vi "Put Object from file (Multipart).vi"(4 "Region":T1, 6 "Chunk size (kB)":i32=5120 min=5120, 7 "Request Parameters":T3={"Content Type"="binary/octet-stream", "ACL"=enum."private", "Storage Class"=enum."STANDARD", "User Metadata"=[]}, 8 "error in (no error)":errorcluster, 9 "Bucket":string, 10 "Object Path":string, 11 "Local file path":path) -> (0 "error out":errorcluster, 2 "Version ID":string, 3 "CompleteMultipartUploadResult":T2)   [LabVIEW 2015, in "LV Interface for Amazon S3.lvlib"]
doc: "This operation <B>uploads an object from a file</B> to a bucket <B>in multiple parts</B>. You can <B>set Chunk size (kB) to limit memory usage</B> of the operation."
uses:
  LV Interface for Amazon S3.lvlib
  Typedefs/AMZ_S3_API_POST Multipart Object Request Parameters.ctl
  Typedefs/AMZ_S3_ACL.ctl
  Typedefs/AMZ_S3_Storage Class.ctl
  Typedefs/AMZ_S3_Object Metadata.ctl
  Typedefs/AMZ_S3_API_CompleteMultipartUploadResult.ctl
  Typedefs/AMZ_S3_LocationConstraint.ctl
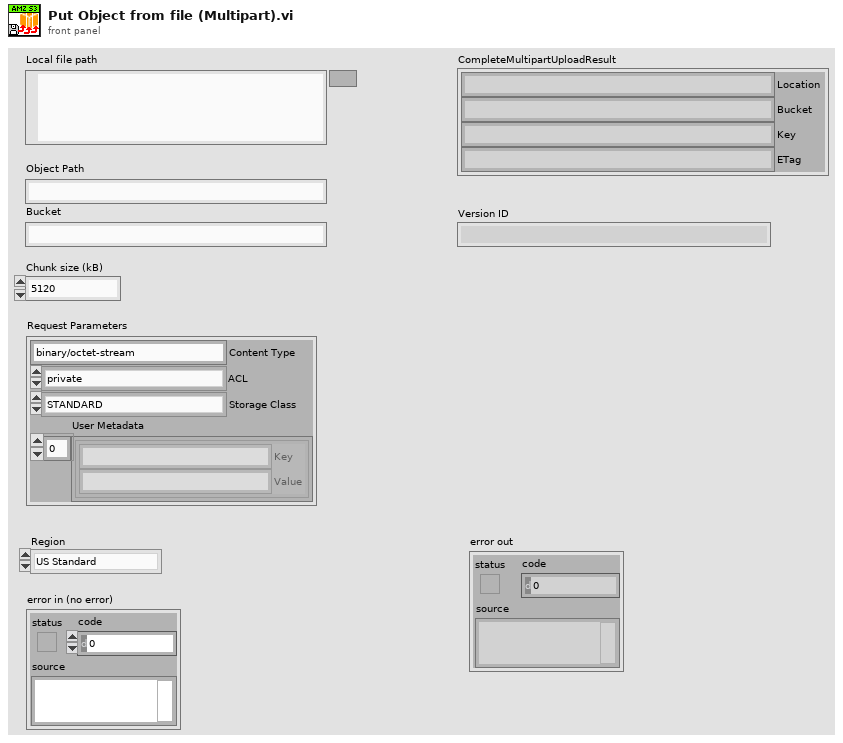
[diagram p1: front panel]
types:
  T1 = typedef "LV Interface for Amazon S3.lvlib/AMZ_S3_LocationConstraint.ctl" = enum16{"US Standard", "us-east-2", "us-west-1", "us-west-2", "ap-northeast-1", "ap-northeast-2", "ap-southeast-1", "ap-southeast-2", "ca-central-1", "eu-central-1", "eu-west-1", "eu-west-2", "sa-east-1"}
  T2 = typedef "LV Interface for Amazon S3.lvlib/AMZ_S3_API_CompleteMultipartUploadResult.ctl" = cluster{"Location":string, "Bucket":string, "Key":string, "ETag":string}
  T3 = typedef "LV Interface for Amazon S3.lvlib/AMZ_S3_API_POST Multipart Object Request Parameters.ctl" = cluster{"Content Type":string, "ACL":T4, "Storage Class":T5, "User Metadata":T6[]}
  T4 = typedef "LV Interface for Amazon S3.lvlib/AMZ_S3_ACL.ctl" = enum16{"private", "public-read", "public-read-write", "aws-exec-read", "authenticated-read", "bucket-owner-read", "bucket-owner-full-control"}
  T5 = typedef "LV Interface for Amazon S3.lvlib/AMZ_S3_Storage Class.ctl" = enum16{"STANDARD", "REDUCED_REDUNDANCY"}
  T6 = typedef "LV Interface for Amazon S3.lvlib/AMZ_S3_Object Metadata.ctl" = cluster{"Key":string, "Value":string}
  T7 = typedef "LV Interface for Amazon S3.lvlib/AMZ_S3_Multipart Upload RefNum.ctl" = refnum<k1>
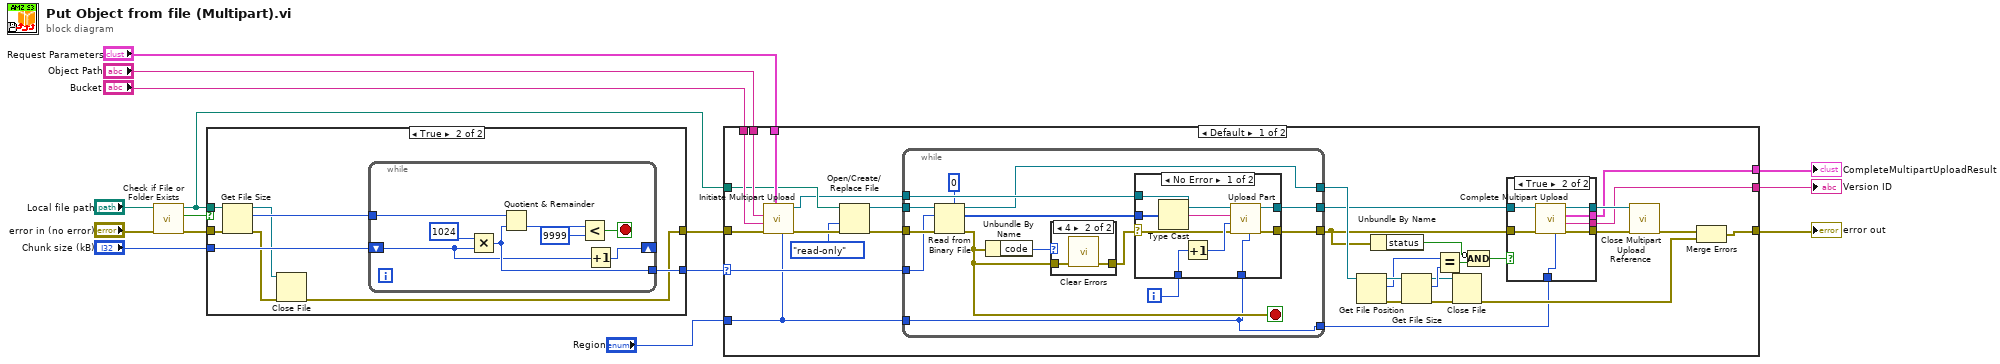
[diagram p0: block diagram]
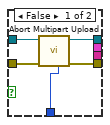
[diagram p2: hidden frame]
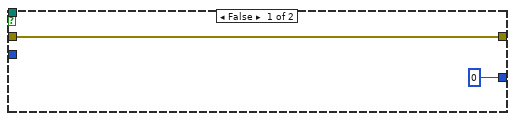
[diagram p6: hidden frame]
diagram:
  n1 = call <vilib>:"Check if File or Folder Exists.vi"("error in (no error)"="error in (no error)", "path"="Local file path") -> ("error out"=w12:errorcluster, "file or folder exists?"=w13:bool, "dup path"=w5:path)  [unwired: 7 in]
  n2 = case shown="True" w13 {
    tunnel: w12 -> [w16 w24]
    tunnel: w5 -> [_ w25]
    tunnel: "Chunk size (kB)" -> [_ w23]
    tunnel: [0 w21] -> w10
    tunnel: [w16 w19] -> w9
    frame False {
    }
    frame True {
      n3 = Get File Size(file=w25, error in=w24) -> (refnum out=w18:refnum<file>, size (in bytes)=w22:i64, 0:w20:errorcluster)
      n4 = Close File(refnum=w18, error in=w20) -> (error out=w19:errorcluster)  [unwired: 1 out]
      n5 = while {
        tunnel: w22 -> [w33]
        shift-right: [w27] -> _
        shift-left: w23 -> [w26]
        tunnel: [w28] -> w21
        stop <- w30 stop-if-true
        n6 = Multiply(x=1024 ("y"), y=w26) -> (x*y=w28:i32)
        n7 = Quotient & Remainder(x=w33, y=w28) -> (floor(x/y)=w32:i64)  [unwired: 1 out]
        n8 = Less?(x=w32, y=i64 9999) -> (x < y?=w30:bool)
        n9 = Increment(x=w26) -> (x+1=w27:i32)
      }
    }
  }
  n10 = case shown="Default" w10 {
    selector: w10 -> [w36 _]
    tunnel: w9 -> [w62 w106]
    tunnel: "Bucket" -> [w65 _]
    tunnel: "Object Path" -> [w64 _]
    tunnel: "Request Parameters" -> [w63 _]
    tunnel: w5 -> [w60 _]
    tunnel: [w38 w106] -> w3
    tunnel: [w41 _] -> w4
    tunnel: [w37 _] -> w2
    tunnel: "Region" -> [w34 _]
    frame Default {
      n11 = call "Initiate Multipart Upload.vi"("Region"=w34, "Request Parameters"=w63, "error in (no error)"=w62, "Bucket"=w65, "Object Path"=w64) -> ("error out"=w61:errorcluster, "Multipart Upload RefNum"=w59:T7)  [unwired: 5 in]
      n12 = Open/Create/Replace File(file path (use dialog)=w60, error in=w61, access (0:read/write)=enum16{"read/write", "read-only", "write-only"}."read-only") -> (refnum out=w56:refnum<file>, error out=w57:errorcluster)  [unwired: 3 in, 1 out]
      n13 = while {
        tunnel: w57 -> [w91]
        tunnel: w56 -> [w90]
        tunnel: w59 -> [w89]
        tunnel: [w80] -> w44
        tunnel: [w79] -> w51
        tunnel: [w88] -> w46
        tunnel: w36 -> [w84]
        tunnel: w34 -> [w78]
        tunnel: [w78] -> w35
        i -> [w87]
        stop <- w81 stop-if-true
        n14 = Read from Binary File(5:u8 0, 8:w91, 10:w84, 11:w90) -> (0:w81:errorcluster, 2:w85:u8[], 3:w79:refnum<file>)  [unwired: 2 in, 1 out]
        n15 = Unbundle By Name(w81) -> ("code"=w83:i32)
        n16 = case shown="4" w83 {
          tunnel: w81 -> [w103 w105]
          tunnel: [w103 w104] -> w82
          frame Default {
          }
          frame 4 {
            n17 = call <vilib>:"Clear Errors.vi"("error in (no error)"=w105) -> ("error out"=w104:errorcluster)  [unwired: 5 in, 1 out]
          }
        }
        n18 = case shown="No Error" w82 {
          selector: w82 -> [w94 w102]
          tunnel: w89 -> [w100 w101]
          tunnel: [w99 w101] -> w88
          tunnel: w87 -> [w98 _]
          tunnel: w85 -> [w96 _]
          tunnel: [w93 w102] -> w80
          tunnel: w78 -> [w92 _]
          frame No Error {
            n19 = Type Cast(x=w96) -> (*(type *) &x=w95:string)  [unwired: 1 in]
            n20 = Increment(x=w98) -> (x+1=w97:i32)
            n21 = call "Upload Part.vi"("Region"=w92, "error in (no error)"=w94, "Part Number"=w97, "Data"=w95, "Multipart Upload RefNum in"=w100) -> ("error out"=w93:errorcluster, "Multipart Upload RefNum out"=w99:T7)  [unwired: 4 in, 1 out]
          }
          frame Error {
          }
        }
      }
      n22 = Get File Position(7:w51) -> (0:w54:errorcluster, 2:w52:i64, 3:w55:refnum<file>)  [unwired: 1 in]
      n23 = Unbundle By Name(w44) -> ("status"=w48:bool)
      n24 = Get File Size(file=w55, error in=w54) -> (refnum out=w49:refnum<file>, size (in bytes)=w53:i64, 0:w50:errorcluster)
      n25 = Equal?(x=w52, y=w53) -> (x = y?=w47:bool)
      n26 = Close File(refnum=w49, error in=w50) -> (error out=w39:errorcluster)  [unwired: 1 out]
      n27 = Compound Arithmetic op=AND(invert w48, w47) -> (w45:bool)
      n28 = case shown="True" w45 {
        tunnel: w46 -> [w69 w76]
        tunnel: w44 -> [w70 w77]
        tunnel: [w67 w75] -> w43
        tunnel: [_ w74] -> w41
        tunnel: [w68 w73] -> w42
        tunnel: [_ w72] -> w37
        tunnel: w35 -> [w66 w71]
        frame False {
          n29 = call "Abort Multipart Upload.vi"("Region"=w66, "error in (no error)"=w70, "Multipart Upload RefNum in"=w69) -> ("error out"=w67:errorcluster, "Multipart Upload RefNum out"=w68:T7)  [unwired: 6 in, 1 out]
        }
        frame True {
          n30 = call "Complete Multipart Upload.vi"("Region"=w71, "error in (no error)"=w77, "Multipart Upload RefNum in"=w76) -> ("error out"=w75:errorcluster, "Version ID"=w72:string, "CompleteMultipartUploadResult"=w74:T2, "Multipart Upload RefNum out"=w73:T7)  [unwired: 5 in]
        }
      }
      n31 = call "Close Multipart Upload Reference.vi"("error in (no error)"=w43, "Multipart Upload RefNum in"=w42) -> ("error out"=w40:errorcluster)  [unwired: 9 in]
      n32 = Merge Errors(w40, w39) -> (w38:errorcluster)
    }
    frame 0 {
    }
  }
  "error out" <- w3
  "CompleteMultipartUploadResult" <- w4
  "Version ID" <- w2
